vi "Main.vi"() -> ()   [LabVIEW 2015]
uses:
  TypeDefs/States.ctl
  TypeDefs/Acq Loop Data.ctl
  TypeDefs/Buttons UI.ctl
panel:
  in  "#samples":dbl=100.0
  in  "Frequency":dbl=1000.0
  out "File Path":path
  in  "File Name Prefix":string="LV Academy"
  in  "Buttons":T1
  out "Wykres":dbl[](graph)
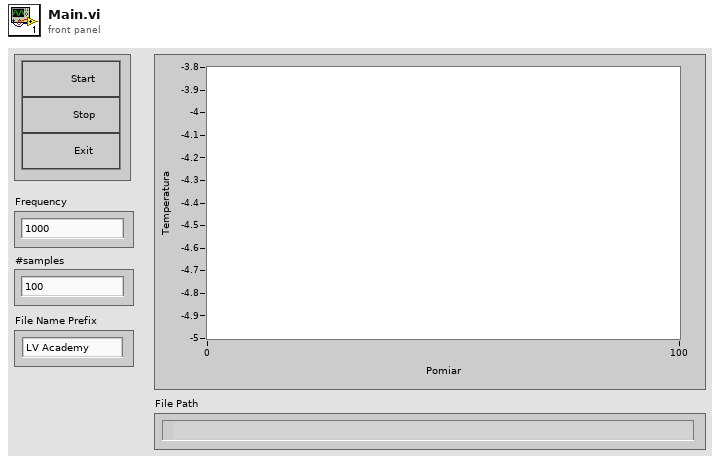
[diagram p1: front panel]
types:
  T1 = typedef "Buttons UI.ctl" = cluster{"Start":bool, "Stop":bool, "Exit":bool}
  T2 = typedef "Acq Loop Data.ctl" = cluster{"File Name Profix":string, "Frequency":dbl, "#samples":i32, "DAQ task ":refnum<k21>}
  T3 = typedef "Queue Data" = cluster{"Action":string, "Data":dbl[]}
  T4 = typedef "States.ctl" = enum16{"Check if Stop or Exit", "Exit", "Wait for Start or Exit", "Start Acquisition", "Reset Acquisition", "Acquisition"}
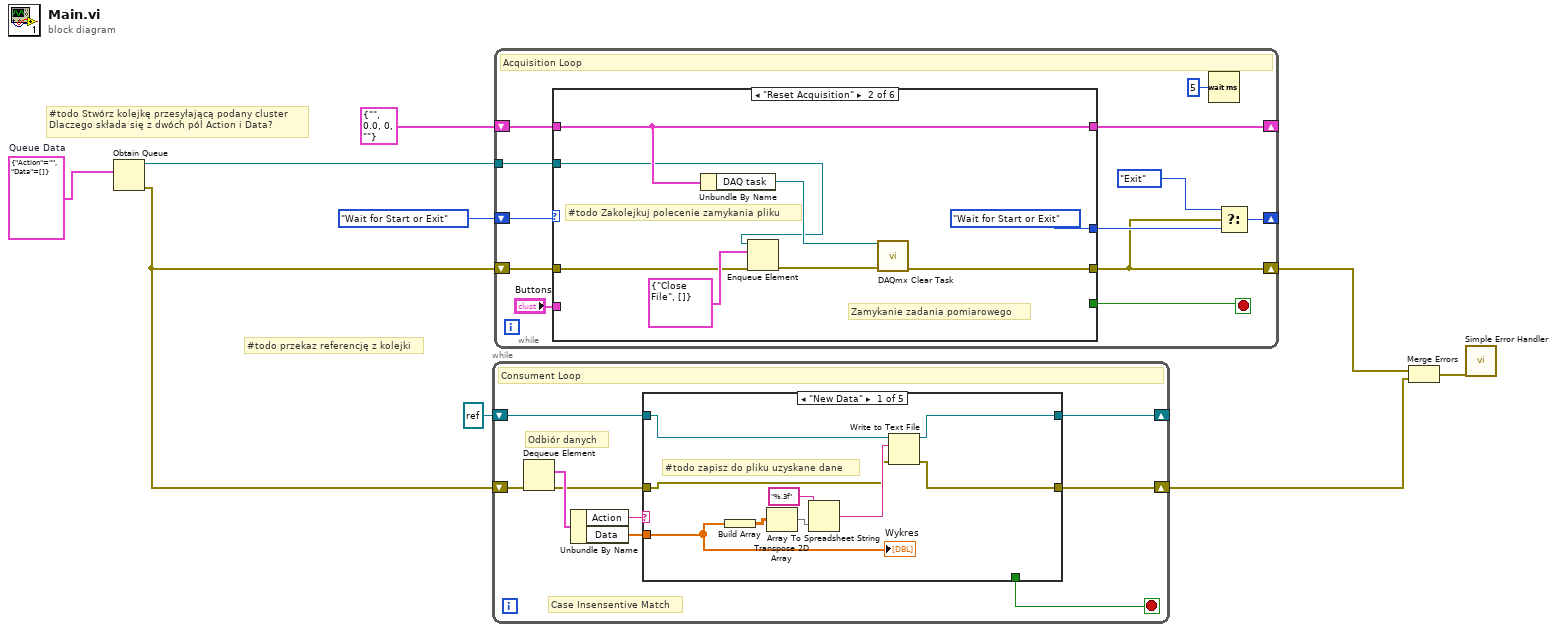
[diagram p0: block diagram]
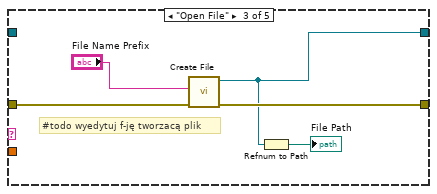
[diagram p3: hidden frame]
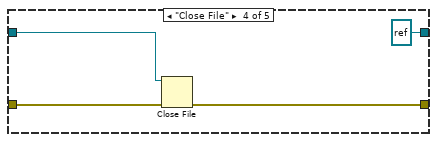
[diagram p4: hidden frame]
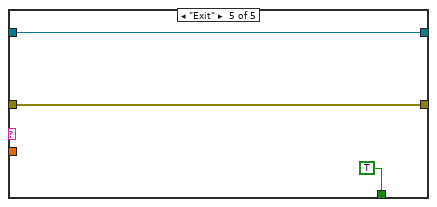
[diagram p5: hidden frame]
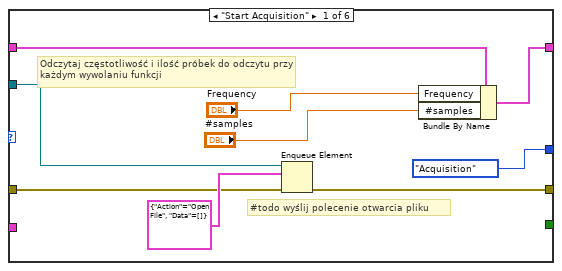
[diagram p6: hidden frame]
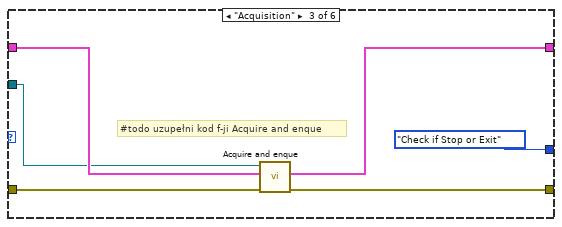
[diagram p7: hidden frame]
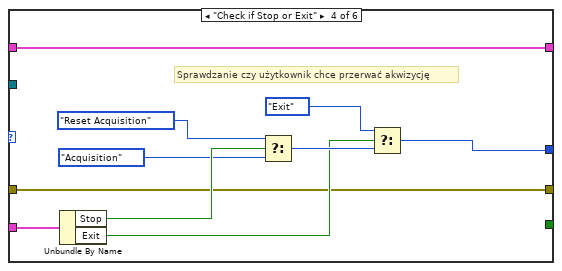
[diagram p8: hidden frame]
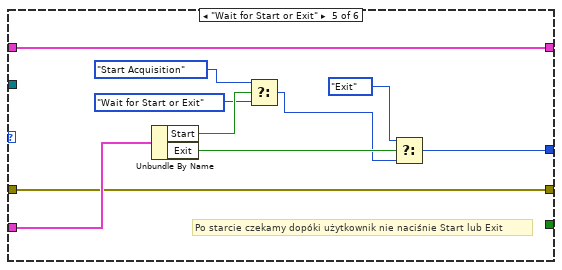
[diagram p9: hidden frame]
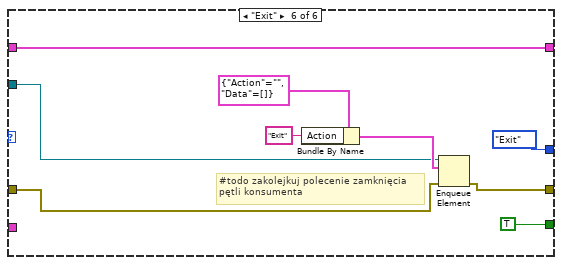
[diagram p10: hidden frame]
diagram:
  w3 = T3 {"Action"="", "Data"=[]}  # Queue Data
  # "#todo przekaz referencję z kolejki"
  # "#todo Stwórz kolejkę przesyłającą podany cluster\nDlaczego składa się z dwóch pól Action i Data?"
  n1 = Obtain Queue(element data type=w3) -> (queue out=w2:refnum<queue>, error out=w1:errorcluster)  [unwired: 4 in, 1 out]
  n2 = while {
    shift-right: [w12] -> w6
    shift-left: w1 -> [w18]
    shift-right: [w13] -> _
    shift-left: refnum<file> refnum ("refnum out") -> [w11]
    stop <- w10 stop-if-true
    # "Odbiór danych"
    # "Case Insensentive Match"
    # "Consument Loop"
    n3 = Dequeue Element(error in (no error)=w18) -> (element=w17:T3, error out=w14:errorcluster)  [unwired: 2 in, 2 out]
    n4 = Unbundle By Name(w17) -> ("Action"=w16:string, "Data"=w15:dbl[])
    n5 = case shown="\"New Data\"" w16 {
      tunnel: w15 -> [w26 _ _ _ _]
      tunnel: w14 -> [w21 w29 w34 w38 w40]
      tunnel: [w19 w28 w30 refnum<file> refnum ("refnum out") w39] -> w13
      tunnel: [w20 w29 w32 w36 w40] -> w12
      tunnel: w11 -> [w27 w28 _ w37 w39]
      tunnel: [_ _ _ _ TRUE] -> w10
      frame "New Data" {
        # "#todo zapisz do pliku uzyskane dane"
        n6 = Build Array(w26) -> (w25:dbl[][])
        n7 = Transpose 2D Array(2D array=w25) -> (transposed array=w24:dbl[][])
        n8 = Array To Spreadsheet String(array=w24, 3:"%.3f" ("format string")) -> (spreadsheet string=w22:string)  [unwired: 1 in]
        n9 = Write to Text File(file (use dialog)=w27, text=w22, error in=w21) -> (refnum out=w19:refnum<file>, error out=w20:errorcluster)  [unwired: 1 in, 1 out]
        "Wykres" <- w26
      }
      frame Default {
      }
      frame "Open File" {
        # "#todo wyedytuj f-ję tworzacą plik"
        n10 = call "Create File.vi"("error in (no error)"=w34, "File Name Prefix"="File Name Prefix") -> ("error out"=w32:errorcluster, "refnum out"=w30:refnum<file>)  [unwired: 8 in]
        n11 = Refnum to Path(1:w30) -> (0:→"File Path":path)
      }
      frame "Close File" {
        n12 = Close File(refnum=w37, error in=w38) -> (error out=w36:errorcluster)  [unwired: 1 out]
      }
      frame "Exit" {
      }
    }
  }
  n13 = while {
    shift-right: [w45] -> _
    shift-left: States."Wait for Start or Exit" -> [w53]
    shift-right: [w49] -> _
    shift-left: T2 {"File Name Profix"="", "Frequency"=0.0, "#samples"=0, "DAQ task "=""} -> [w50]
    shift-right: [w43] -> w5
    shift-left: w1 -> [w52]
    tunnel: w2 -> [w42]
    stop <- w47 stop-if-true
    # "Acquisition Loop"
    n14 = case shown="\"Reset Acquisition\"" w53 {
      tunnel: w52 -> [w55 w65 w76 w78 w89 w98]
      tunnel: "Buttons" -> [_ _ _ w86 w96 _]
      tunnel: [States."Acquisition" States."Wait for Start or Exit" States."Check if Stop or Exit" w79 w91 States."Exit"] -> w46
      tunnel: w50 -> [w62 w67 w75 w77 w90 w102]
      tunnel: [w59 w67 w72 w77 w90 w102] -> w49
      tunnel: [w54 w70 w74 w78 w89 w97] -> w43
      tunnel: [_ _ _ _ _ TRUE] -> w47
      tunnel: w42 -> [w56 w63 w71 _ _ w99]
      frame "Start Acquisition" {
        # "#todo wyślij polecenie otwarcia pliku"
        # "Odczytaj częstotliwość i ilość próbek do odczytu przy każdym wywolaniu funkcji"
        n15 = Enqueue Element(queue=w56, element=T3 {"Action"="Open File", "Data"=[]}, error in (no error)=w55) -> (error out=w54:errorcluster)  [unwired: 1 in, 2 out]
        n16 = Bundle By Name(cluster=w62, "Frequency"="Frequency", "#samples"="#samples") -> (w59:T2)
      }
      frame "Reset Acquisition" {
        # "#todo Zakolejkuj polecenie zamykania pliku"
        # "Zamykanie zadania pomiarowego"
        n17 = Unbundle By Name(w67) -> ("DAQ task"=w69:refnum<k21>)
        n18 = Enqueue Element(queue=w63, element=T3 {"Action"="Close File", "Data"=[]}, error in (no error)=w65) -> (error out=w64:errorcluster)  [unwired: 1 in, 2 out]
        n19 = call <vilib>:"DAQmx Clear Task.vi"("task in"=w69, "error in"=w64) -> ("error out"=w70:errorcluster)  [unwired: 13 in]
      }
      frame "Acquisition" {
        # "#todo uzupełni kod f-ji Acquire and enque"
        n20 = call "Acquire and enque.vi"("error in (no error)"=w76, "Data In"=w75, "Queue in"=w71) -> ("error out"=w74:errorcluster, "Data Out"=w72:T2)  [unwired: 7 in]
      }
      frame "Check if Stop or Exit" {
        # "Sprawdzanie czy użytkownik chce przerwać akwizycję"
        n21 = Unbundle By Name(w86) -> ("Stop"=w85:bool, "Exit"=w81:bool)
        n22 = Select(t=States."Reset Acquisition", s=w85, f=States."Acquisition") -> (s? t:f=w82:T4)
        n23 = Select(t=States."Exit", s=w81, f=w82) -> (s? t:f=w79:T4)
      }
      frame "Wait for Start or Exit" {
        # "Po starcie czekamy dopóki użytkownik nie naciśnie Start lub Exit"
        n24 = Unbundle By Name(w96) -> ("Start"=w95:bool, "Exit"=w92:bool)
        n25 = Select(t=States."Start Acquisition", s=w95, f=States."Wait for Start or Exit") -> (s? t:f=w88:T4)
        n26 = Select(t=States."Exit", s=w92, f=w88) -> (s? t:f=w91:T4)
      }
      frame "Exit" {
        # "#todo zakolejkuj polecenie zamknięcia\npętli konsumenta"
        n27 = Bundle By Name(cluster=T3 {"Action"="", "Data"=[]}, "Action"="Exit") -> (w100:T3)
        n28 = Enqueue Element(queue=w99, element=w100, error in (no error)=w98) -> (error out=w97:errorcluster)  [unwired: 1 in, 2 out]
      }
    }
    n29 = Wait (ms)(milliseconds to wait=u32 5) -> ()  [unwired: 1 out]
    n30 = Select(t=States."Exit", s=w43, f=w46) -> (s? t:f=w45:T4)
  }
  n31 = Merge Errors(w5, w6) -> (w4:errorcluster)
  n32 = call <vilib>:"Simple Error Handler.vi"("error in (no error)"=w4) -> ()  [unwired: 4 in, 5 out]
